vi "Convert Analog.vi"(7 "Input Value":dbl, 8 "Sensor Min":dbl, 9 "Sensor Max":dbl, 10 "Signal Min":dbl, 11 "Signal Max":dbl) -> (3 "result":dbl)   [LabVIEW 2024, in "Hardware Controller.lvlib"]
uses:
  Hardware Controller.lvlib
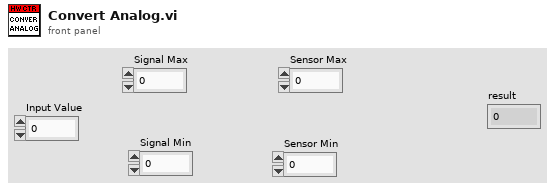
[diagram p1: front panel]
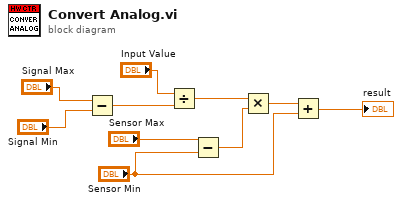
[diagram p0: block diagram]
diagram:
  n1 = Subtract(x="Signal Max", y="Signal Min") -> (x-y=w7:dbl)
  n2 = Divide(x="Input Value", y=w7) -> (x/y=w5:dbl)
  n3 = Subtract(x="Sensor Max", y="Sensor Min") -> (x-y=w4:dbl)
  n4 = Multiply(x=w5, y=w4) -> (x*y=w3:dbl)
  n5 = Add(x=w3, y="Sensor Min") -> (x+y=→"result":dbl)
